vi "test Request Response.vi"(8 "error in (no error)":errorcluster, 11 "TestCase in":refnum<class "Message Test Case.lvclass">) -> (0 "error out":errorcluster, 3 "TestCase out":refnum<class "Message Test Case.lvclass">)   [LabVIEW 2027, in "Message Test Case.lvclass"]
uses:
  Message Test Case.lvclass
  Consumer/Abstract Consumer/Abstract Consumer.lvclass
  Support/Messages/Count Response Message/Count Response Message.lvclass
  Support/Messages/Count Response Message/Count Response Message.lvclass/Count Response Message.ctl
  Support/Messages/Count Response Message/Read Count.vi
  Support/Messages/Count Request Message/Count Request Message.lvclass
  C:/Program Files/National Instruments/LabVIEW 2027/vi.lib/addons/_JKI Toolkits/VI Tester/TestCase.llb/TestCase.lvclass
  <vilib>/addons/_JKI Toolkits/VI Tester/TestCase.llb/TestCase.lvclass
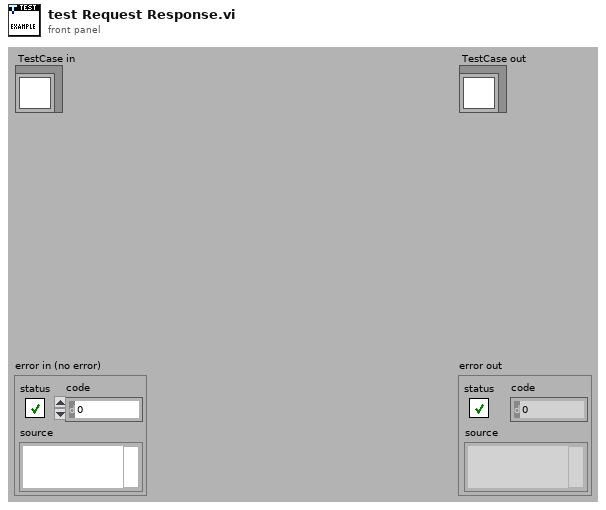
[diagram p1: front panel]
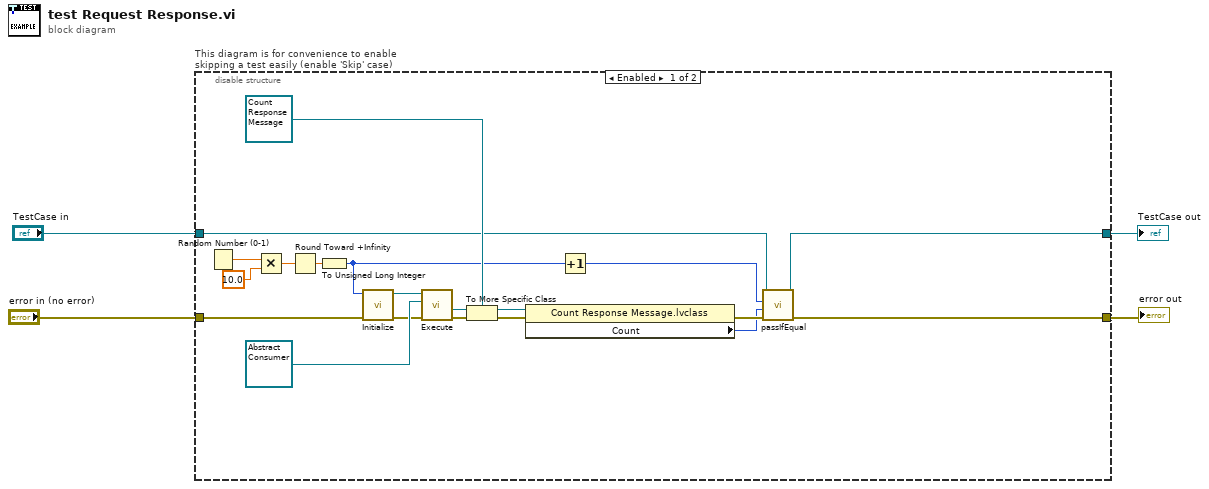
[diagram p0: block diagram]
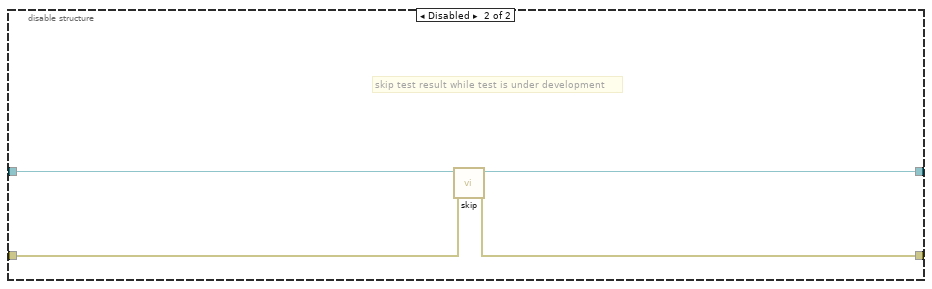
[diagram p2: hidden frame]
diagram:
  n1 = disable-structure "This diagram is for convenience to enable skipping a test easily (enable 'Skip' case)" shown="Enabled" {
    disable-tunnel: "TestCase in" -> [w17 w28]
    disable-tunnel: [w16 w26] -> w1
    disable-tunnel: [w14 w27] -> w3
    disable-tunnel: "error in (no error)" -> [w13 w25]
    frame Enabled {
      n2 = Random Number (0-1)() -> (number: 0 to 1=w10:dbl)
      n3 = Multiply(x=w10, y=10.0) -> (x*y=w8:dbl)
      n4 = Round Toward +Infinity(x=w8) -> (ceil(x): smallest int >= x=w7:dbl)
      n5 = To Unsigned Long Integer(number=w7) -> (unsigned 32bit integer=w6:u32)
      n6 = call "Initialize.vi"("error in (no error)"=w13, "Initial Count (0)"=w6) -> ("error out"=w12:errorcluster, "Count Request Message out"=w11:refnum<class "Count Request Message.lvclass">)  [unwired: 8 in]
      n7 = call-dynamic "Execute.vi"("error in (no error)"=w12, "Abstract Consumer in"=refnum<class "Abstract Consumer.lvclass"> refnum, "Count Request Message in"=w11) -> ("error out"=w23:errorcluster, "Abstract Response out"=w22:refnum<class "Abstract Response Message.lvclass">)  [unwired: 4 in, 3 out]
      n8 = To More Specific Class(target class=refnum<class "Count Response Message.lvclass"> refnum ("Count Response Message.lvclass"), reference=w22, error in=w23) -> (specific class reference=w20:refnum<class "Count Response Message.lvclass">, error out=w19:errorcluster)
      n9 = property class="Count Response Message.lvclass"(reference=w20, error in=w19) -> (error out=w18:errorcluster, "Count"=w15:u32)  [unwired: 1 out]
      n10 = Increment(x=w6) -> (x+1=w5:u32)
      n11 = call-dynamic "passIfEqual.vi"("error in (no error)"=w18, "y"=w15, "x"=w5, "TestCase in"=w17) -> ("error out"=w14:errorcluster, "TestCase out"=w16:refnum<class "Message Test Case.lvclass">)  [unwired: 6 in]
    }
    frame Disabled {
      # "skip test result while test is under development"
      n12 = call <vilib>:"skip.vi"("error in (no error)"=w25, "TestCase in"=w28) -> ("error out"=w27:errorcluster, "TestCase out"=w26:refnum<class "Message Test Case.lvclass">)  [unwired: 8 in]
    }
  }
  "error out" <- w3
  "TestCase out" <- w1
